vi "array -- linear regression 2D -- V2.vi"(7 "action":T2, 9 "fit map IN":map{T1, dbl}(c390), 11 "xyz IN":cluster{"x":dbl[], "y":dbl[], "z":dbl[]}={"x"=[0.0, 0.0, 0.0, -1.0, -1.0, -1.0, 1.0, 1.0, 1.0], "y"=[-1.0, 0.0, 1.0, -1.0, 0.0, 1.0, -1.0, 0.0, 1.0], "z"=[1.0, 0.0, 1.0, 4.0, 1.0, 0.0, 0.0, 1.0, 4.0]}) -> (1 "fit map out":map{T1, dbl}(c390), 3 "xyz OUT":cluster{"x":dbl[], "y":dbl[], "z":dbl[]}={"x"=[0.0, 0.0, 0.0, -1.0, -1.0, -1.0, 1.0, 1.0, 1.0], "y"=[-1.0, 0.0, 1.0, -1.0, 0.0, 1.0, -1.0, 0.0, 1.0], "z"=[1.0, 0.0, 1.0, 4.0, 1.0, 0.0, 0.0, 1.0, 4.0]})   [LabVIEW 2021]
uses:
  array -- fit control .ctl
  array -- bilinear regression 2D.ctl
  <vilib>/Analysis/baseanly.llb/Matrix Type of Inverse Matrix.ctl
  <vilib>/Analysis/7linalg.llb/Solve Linear Equations (single right hand).vi
  <vilib>/Analysis/baseanly.llb/Solve Linear Equations By Cholesky.vi
  <vilib>/Analysis/baseanly.llb/Real Matrix to Compact Array.vi
  <vilib>/Analysis/baseanly.llb/Real Compact Tri-Matrix Linear Eqs.vi
  <vilib>/Analysis/Matrix/Numeric/Conversions/Array To Matrix - RA2.vi
  <vilib>/Analysis/7linalg.llb/Solve Linear Eqs (General).vi
  <vilib>/Analysis/7linalg.llb/Solve Linear Eqs (Gen, single right hand).vi
  <vilib>/Analysis/Matrix/NI_Matrix.lvlib
  <vilib>/Analysis/NI_AALPro.lvlib
  <vilib>/Analysis/NI_AALBase.lvlib
panel:
  out "fit  out":dbl[](array[numeric])=[1.9, 2.6, 3.3, 1.0, 2.7, 3.9]
  out "fit  IN":dbl[](array[numeric])=[1.9, 2.6, 3.3, 1.0, 2.7, 3.9]
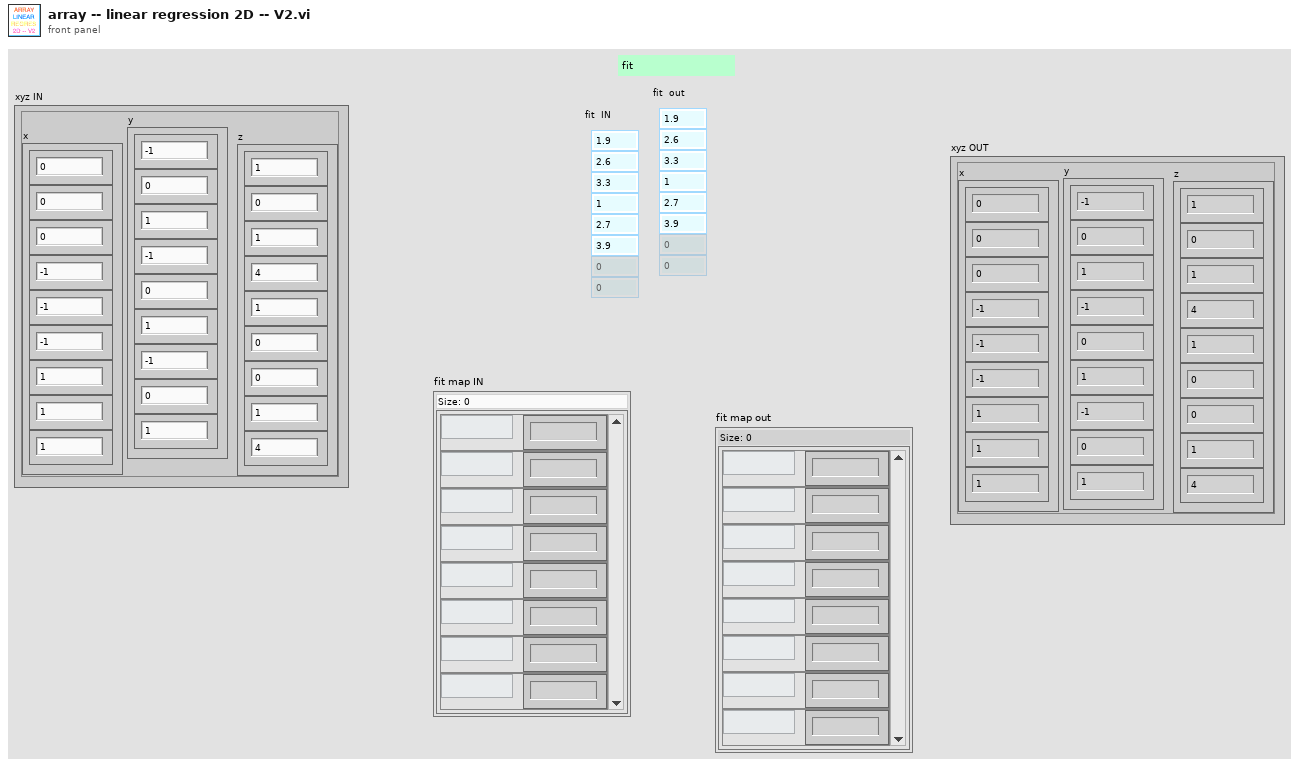
[diagram p1: front panel]
types:
  T1 = typedef "array -- bilinear regression 2D.ctl" = enum16{"1", "x", "y", "xx", "xy", "yy", "xxy", "xyy", "yyy", "xxx", "xxyy", "xyyy", "xxxy", "yyyy", "xxxx", "xxz", "xyz", "yyz", "xz", "yz", "z", "wwz", "ywz", "xwz", "xxxw", "xxyw", "xyyw", "yyyw", "xxww", "xyww", "yyww", "xwww", "ywww", "wwww", "ww", "xw", "yw", "w", "wz"}
  T2 = typedef "array -- fit control .ctl" = enum16{"fit", "calc", "check", "init"}
  T3 = typedef "NI_AALBase.lvlib/Matrix Type of Inverse Matrix.ctl" = enum32{"General", "Positive Definite", "Lower Triangular", "Upper Triangular"}
  T4 = typedef "NI_Matrix.lvlib/RealMatrix.ctl" = dbl[][]
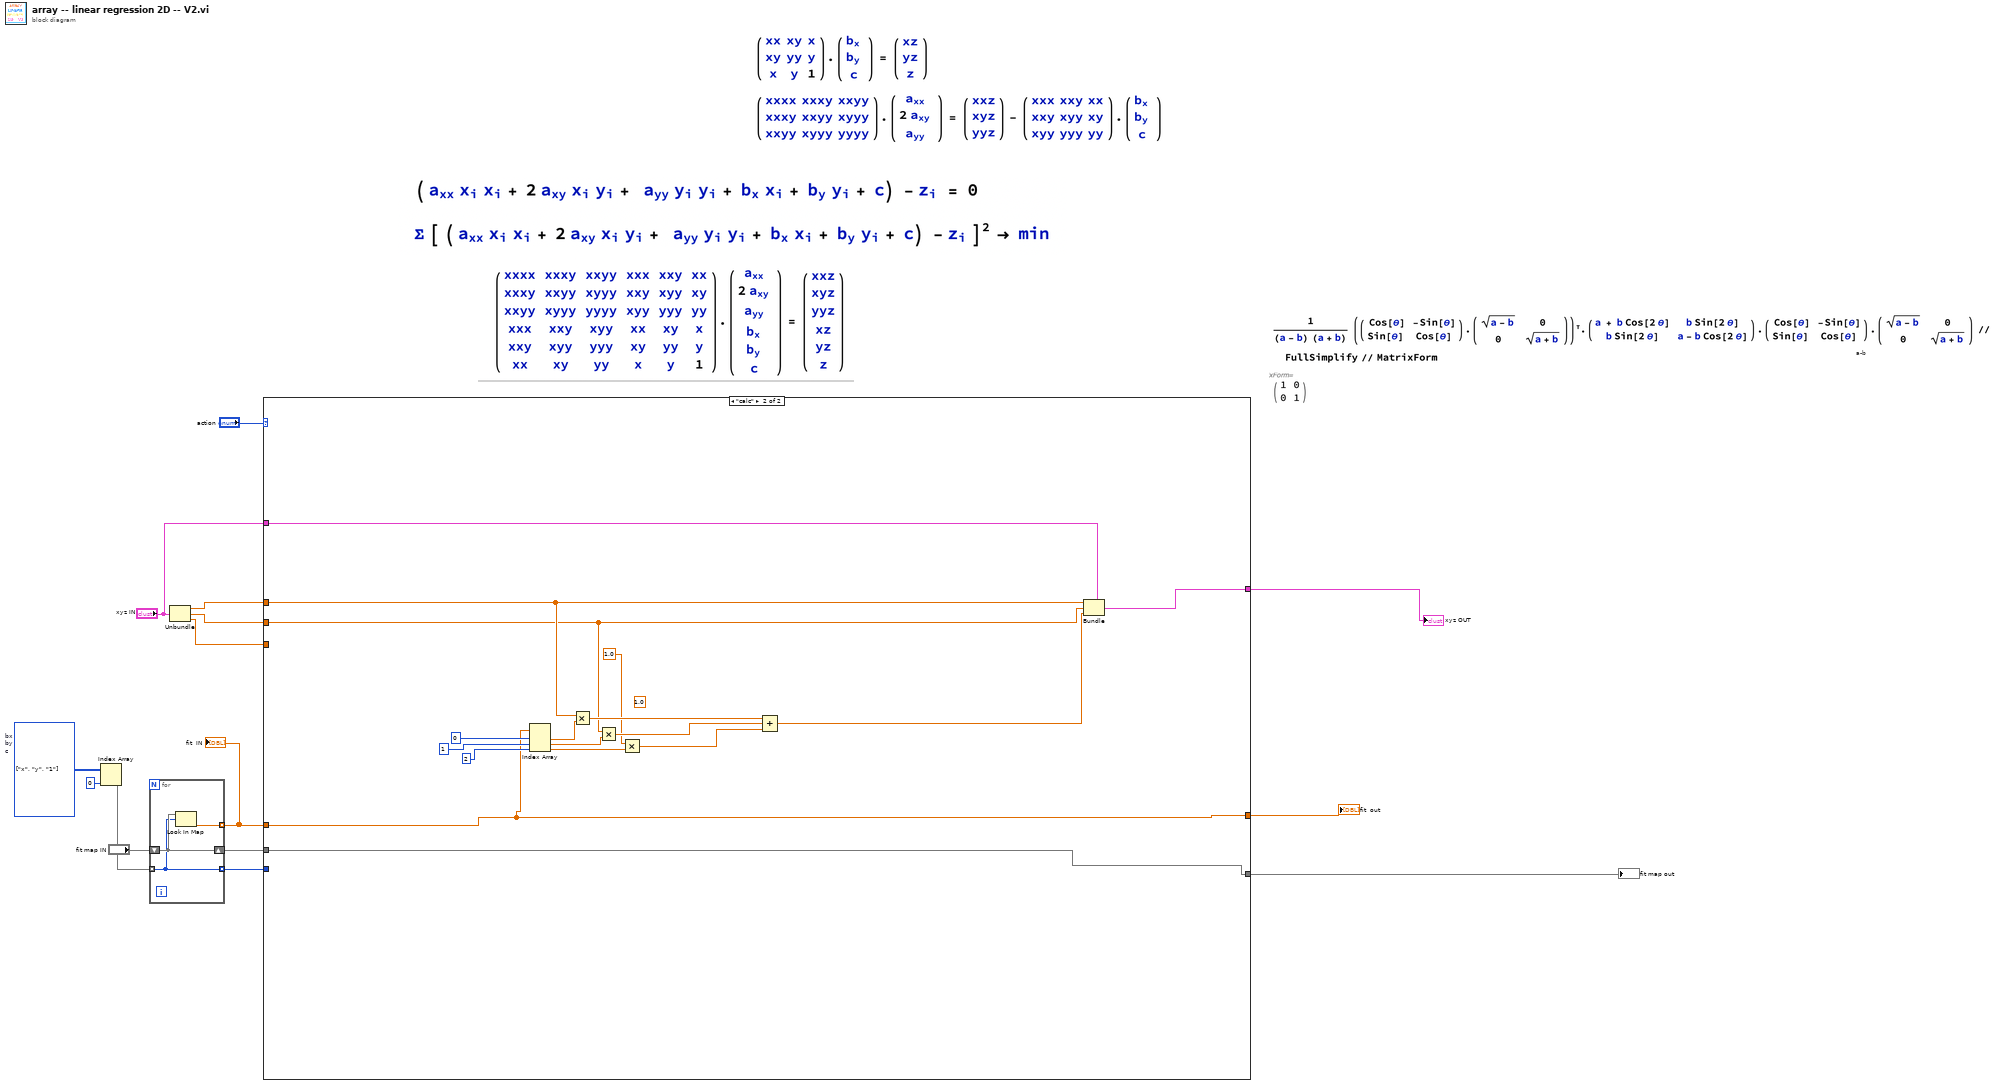
[diagram p0: block diagram]
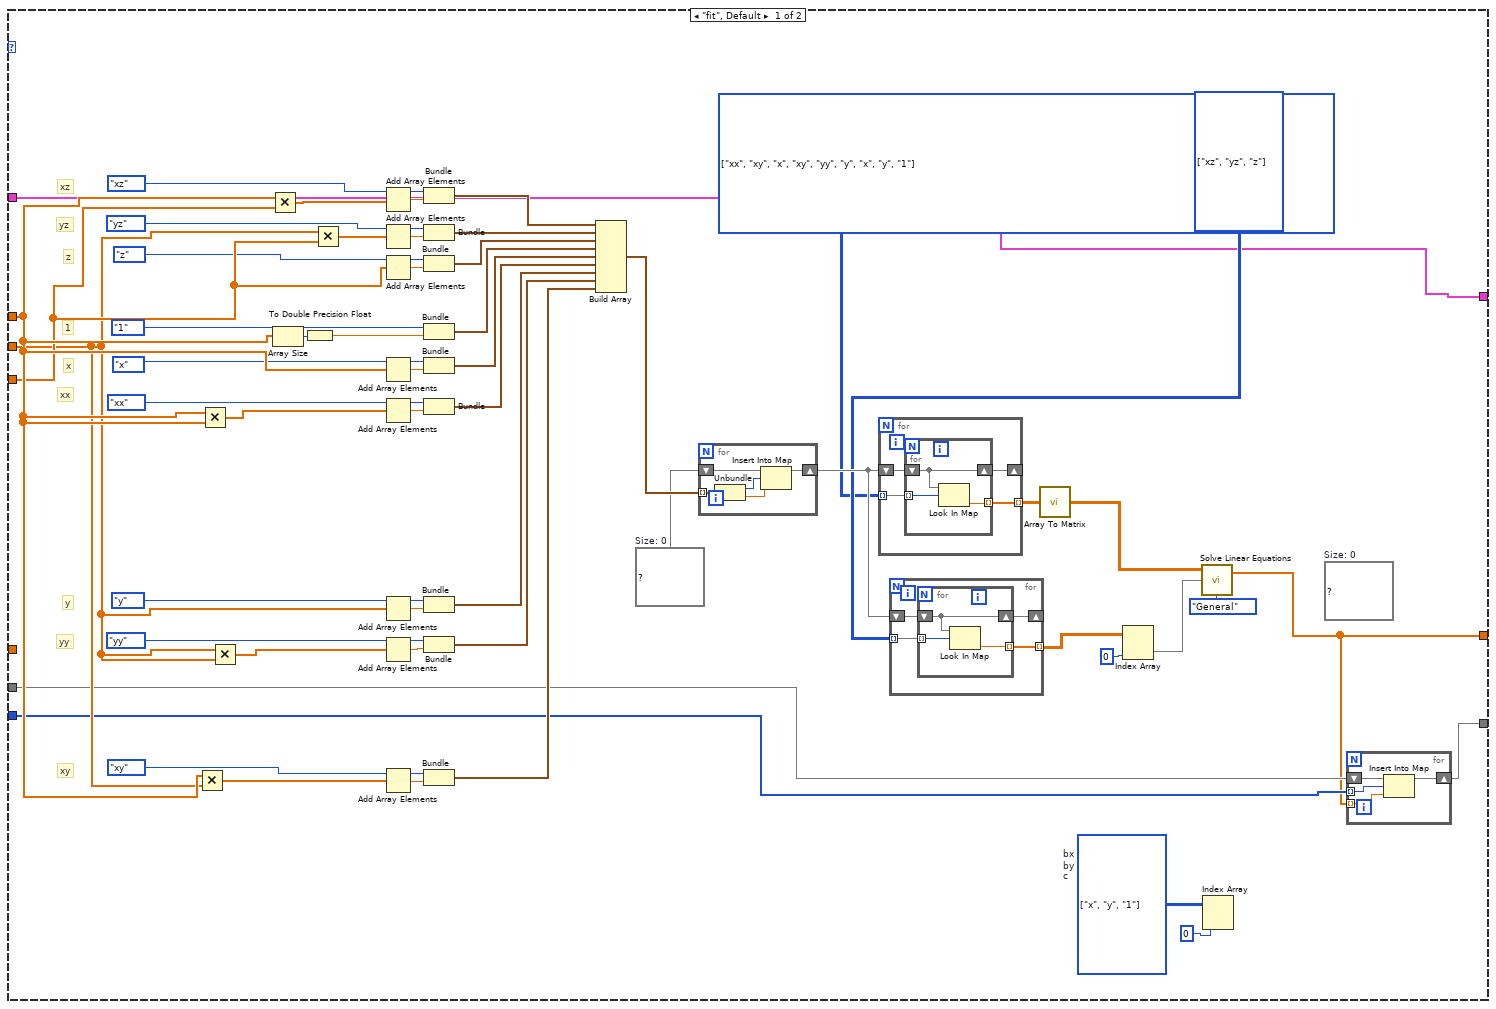
[diagram p2: hidden frame]
diagram:
  w11 = T1[][] [[enum."x"], [enum."y"], [enum."1"]] items=["1", "x", "y", "xx", "xy", "yy", "xxy", "xyy", "yyy", "xxx", "xxyy", "xyyy", "xxxy", "yyyy", "xxxx", "xxz", "xyz", "yyz", "xz", "yz", "z", "wwz", "ywz", "xwz", "xxxw", "xxyw", "xyyw", "yyyw", "xxww", "xyww", "yyww", "xwww", "ywww", "wwww", "ww", "xw", "yw", "w", "wz"]  # bx by c
  # "a-b"
  n1 = Index Array(array=w11, index (col)=0 ("disabled index (col)")) -> (element=w9:T1[])  [unwired: 1 in]
  n2 = for {
    tunnel: w9 -> [w16] mode=indexing
    shift-right: [w18] -> w5
    shift-left: "fit map IN" -> [w18]
    tunnel: [w17] -> w7 mode=indexing
    tunnel: [w16] -> w4 mode=indexing
    n3 = Look In Map(map=w18, key=w16) -> (value=w17:dbl)  [unwired: 1 in, 1 out]
  }
  "fit  IN" <- w7
  n4 = Unbundle("xyz IN") -> ("x"=w14:dbl[], "y"=w13:dbl[], "z"=w12:dbl[])
  n5 = case shown="\"calc\"" "action" {
    tunnel: w12 -> [w68 _]
    tunnel: w14 -> [w71 w100]
    tunnel: [w20 w97] -> w2
    tunnel: w7 -> [_ w97]
    tunnel: w13 -> [w63 w99]
    tunnel: [w28 w112] -> w6
    tunnel: w5 -> [w27 w112]
    tunnel: w4 -> [w26 _]
    tunnel: [w19 w110] -> w3
    tunnel: "xyz IN" -> [w19 w111]
    frame "fit", Default {
      (unwired) map{T1, dbl} {}  # Size: 0
      w30 = T1[][] [[enum."x"], [enum."y"], [enum."1"]] items=["1", "x", "y", "xx", "xy", "yy", "xxy", "xyy", "yyy", "xxx", "xxyy", "xyyy", "xxxy", "yyyy", "xxxx", "xxz", "xyz", "yyz", "xz", "yz", "z", "wwz", "ywz", "xwz", "xxxw", "xxyw", "xyyw", "yyyw", "xxww", "xyww", "yyww", "xwww", "ywww", "wwww", "ww", "xw", "yw", "w", "wz"]  # bx by c
      w34 = T1[][] [[enum."xz"], [enum."yz"], [enum."z"]] items=["1", "x", "y", "xx", "xy", "yy", "xxy", "xyy", "yyy", "xxx", "xxyy", "xyyy", "xxxy", "yyyy", "xxxx", "xxz", "xyz", "yyz", "xz", "yz", "z", "wwz", "ywz", "xwz", "xxxw", "xxyw", "xyyw", "yyyw", "xxww", "xyww", "yyww", "xwww", "ywww", "wwww", "ww", "xw", "yw", "w", "wz"]
      w33 = T1[][] [[enum."xx", enum."xy", enum."x"], [enum."xy", enum."yy", enum."y"], [enum."x", enum."y", enum."1"]] items=["1", "x", "y", "xx", "xy", "yy", "xxy", "xyy", "yyy", "xxx", "xxyy", "xyyy", "xxxy", "yyyy", "xxxx", "xxz", "xyz", "yyz", "xz", "yz", "z", "wwz", "ywz", "xwz", "xxxw", "xxyw", "xyyw", "yyyw", "xxww", "xyww", "yyww", "xwww", "ywww", "wwww", "ww", "xw", "yw", "w", "wz"]
      w36 = map{T1, dbl} {}  # Size: 0
      # "z"
      # "yz"
      # "xz"
      # "xy"
      # "yy"
      # "y"
      # "1"
      # "xx"
      # "x"
      n6 = Multiply(x=w71, y=w63) -> (x*y=w32:dbl[])
      n7 = Multiply(x=w71, y=w71) -> (x*y=w69:dbl[])
      n8 = Multiply(x=w63, y=w63) -> (x*y=w70:dbl[])
      n9 = Multiply(x=w71, y=w68) -> (x*y=w67:dbl[])
      n10 = Array Size(array=w71) -> (size(s)=w56:i32)
      n11 = To Double Precision Float(number=w56) -> (double precision float=w44:dbl)
      n12 = Multiply(x=w63, y=w68) -> (x*y=w72:dbl[])
      n13 = Add Array Elements(numeric array=w67) -> (sum=w53:dbl)
      n14 = Add Array Elements(numeric array=w72) -> (sum=w51:dbl)
      n15 = Add Array Elements(numeric array=w68) -> (sum=w49:dbl)
      n16 = Add Array Elements(numeric array=w71) -> (sum=w58:dbl)
      n17 = Add Array Elements(numeric array=w69) -> (sum=w59:dbl)
      n18 = Add Array Elements(numeric array=w63) -> (sum=w62:dbl)
      n19 = Add Array Elements(numeric array=w70) -> (sum=w64:dbl)
      n20 = Add Array Elements(numeric array=w32) -> (sum=w40:dbl)
      n21 = Bundle(array_--_bilinear_regression_2D."xz", "Numeric"=w53) -> (w48:cluster{T1, "Numeric":dbl})  [unwired: 1 in]
      n22 = Bundle(array_--_bilinear_regression_2D."yz", "Numeric"=w51) -> (w47:cluster{T1, "Numeric":dbl})  [unwired: 1 in]
      n23 = Bundle(array_--_bilinear_regression_2D."z", "Numeric"=w49) -> (w46:cluster{T1, "Numeric":dbl})  [unwired: 1 in]
      n24 = Bundle(array_--_bilinear_regression_2D."1", w44) -> (w45:cluster{T1, dbl})  [unwired: 1 in]
      n25 = Bundle(array_--_bilinear_regression_2D."x", "Numeric"=w58) -> (w43:cluster{T1, "Numeric":dbl})  [unwired: 1 in]
      n26 = Bundle(array_--_bilinear_regression_2D."xx", "Numeric"=w59) -> (w42:cluster{T1, "Numeric":dbl})  [unwired: 1 in]
      n27 = Bundle(array_--_bilinear_regression_2D."y", "Numeric"=w62) -> (w41:cluster{T1, "Numeric":dbl})  [unwired: 1 in]
      n28 = Bundle(array_--_bilinear_regression_2D."yy", "Numeric"=w64) -> (w37:cluster{T1, "Numeric":dbl})  [unwired: 1 in]
      n29 = Bundle(array_--_bilinear_regression_2D."xy", "Numeric"=w40) -> (w31:cluster{T1, "Numeric":dbl})  [unwired: 1 in]
      n30 = Build Array(w48, w47, w46, w45, w43, w42, w41, w37, w31) -> (w39:cluster{T1, "Numeric":dbl}[])
      n31 = for {
        tunnel: w39 -> [w86] mode=indexing
        shift-right: [w87] -> w35
        shift-left: w36 -> [w88]
        n32 = Unbundle(w86) -> (w85:T1, "Numeric"=w84:dbl)
        n33 = Insert Into Map(map in=w88, key=w85, value=w84) -> (map out=w87:map{T1, dbl})  [unwired: 2 out]
      }
      n34 = for {
        tunnel: w33 -> [w92] mode=indexing
        shift-right: [w90] -> _
        shift-left: w35 -> [w91]
        tunnel: [w89] -> w38 mode=indexing
        n35 = for {
          tunnel: w92 -> [w94] mode=indexing
          shift-right: [w95] -> w90
          shift-left: w91 -> [w95]
          tunnel: [w93] -> w89 mode=indexing
          n36 = Look In Map(map=w95, key=w94) -> (value=w93:dbl)  [unwired: 1 in, 1 out]
        }
      }
      n37 = for {
        shift-right: [w79] -> _
        shift-left: w35 -> [w80]
        tunnel: w34 -> [w78] mode=indexing
        tunnel: [w77] -> w22 mode=indexing
        n38 = for {
          shift-right: [w83] -> w79
          shift-left: w80 -> [w83]
          tunnel: w78 -> [w82] mode=indexing
          tunnel: [w81] -> w77 mode=indexing
          n39 = Look In Map(map=w83, key=w82) -> (value=w81:dbl)  [unwired: 1 in, 1 out]
        }
      }
      n40 = call-poly <vilib>:"Array To Matrix.vi"("Real 2D Array"=w38) -> ("Real Matrix"=w21:T4)
      n41 = Index Array(array=w22, index (col)=0 ("disabled index (col)")) -> (element=w24:dbl[])  [unwired: 1 in]
      n42 = call-poly <vilib>:"Solve Linear Equations.vi"("matrix type"=Matrix_Type_of_Inverse_Matrix."General", "Known Vector"=w24, "Input Matrix"=w21) -> ("Solution Vector"=w20:dbl[])  [unwired: 1 out]
      n43 = Index Array(array=w30, index (col)=0 ("disabled index (col)")) -> ()  [unwired: 1 in, 1 out]
      n44 = for {
        shift-right: [w75] -> w28
        shift-left: w27 -> [w76]
        tunnel: w26 -> [w74] mode=indexing
        tunnel: w20 -> [w73] mode=indexing
        n45 = Insert Into Map(map in=w76, key=w74, value=w73) -> (map out=w75:map{T1, dbl})  [unwired: 2 out]
      }
    }
    frame "calc" {
      (unwired) 1.0 ("x")
      n46 = Index Array(array=w97, index #1=0 ("index"), index #2=1 ("index"), index #3=2 ("index")) -> (element #1=w106:dbl, element #2=w105:dbl, element #3=w104:dbl)
      n47 = Multiply(x=w100, y=w106) -> (x*y=w103:dbl[])
      n48 = Multiply(x=w99, y=w105) -> (x*y=w102:dbl[])
      n49 = Multiply(x=1.0, y=w104) -> (x*y=w101:dbl)
      n50 = Compound Arithmetic op=ADD(w103, w102, w101) -> (w96:dbl[])
      n51 = Bundle(cluster=w111, "x"=w100, "y"=w99, "z"=w96) -> (w110:cluster{"x":dbl[], "y":dbl[], "z":dbl[]})
    }
  }
  "fit map out" <- w6
  "xyz OUT" <- w3
  "fit  out" <- w2
